vi "CSM - Remove Module in Boradcast Registry.vi"(0 "CSM Name":string, 11 "Error in":errorcluster caption="Error in (no error)") -> (4 "CSM Name(dup)":string, 15 "Error out":errorcluster)   [LabVIEW 2017, in "Communicable State Machine.lvlib"]
doc: "-- <b>输入控件</b> --\n- <b>CSM Name</b>:\n\n- <B>error in</B> can accept error information wired from VIs previously called. Use this information to decide if any functionality should be bypassed in the event of errors from other VIs.\n\nRight-click the <B>error in</B> control on the front panel and select <B>Explain Error</B> or <B>Explain Warning</B> from the shortcut menu for more information about the error.\n\n-- <b>输出控件</b> --\n- <b>CSM Name(dup)</b>:\n\n- <b>Error out</b>:\n- <B>error out</B> passes error or warning information out of a VI to be used by other VIs.\n\nRight-click the <B>error out</B> indicator on the front panel and select <B>Explain Error</B> or <B>Explain Warning</B> from the shortcut menu for more information about the error."
uses:
  Communicable State Machine.lvlib
  _Support/FGV-BroadcastRegistry/Operation-BroadcastRegistry.ctl
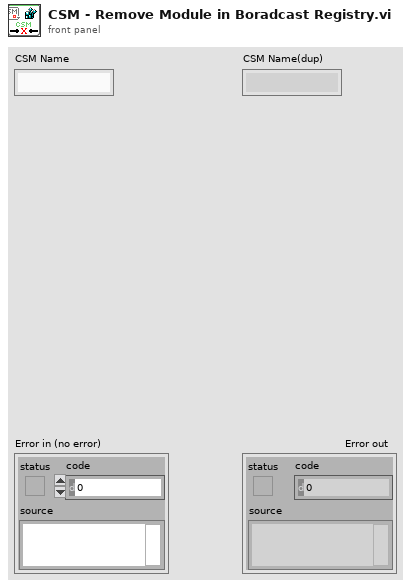
[diagram p1: front panel]
types:
  T1 = typedef "Communicable State Machine.lvlib/Operation-BroadcastRegistry.ctl" = enum16{"Delete Source Module", "Delete Target Module", "Remove Module", "Register", "Unregister", "Check", "List Status", "List Entries"}
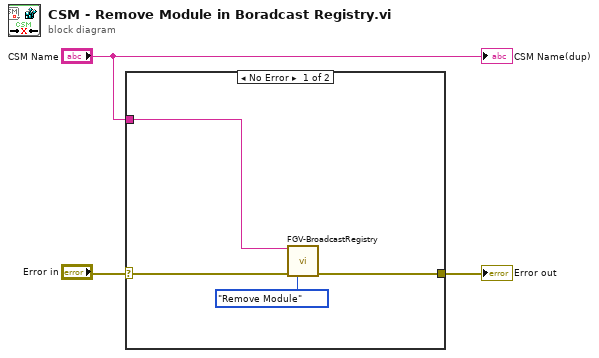
[diagram p0: block diagram]
diagram:
  n1 = case shown="No Error" "Error in" {
    selector: "Error in" -> [w6 w8]
    tunnel: [w5 w8] -> w2
    tunnel: "CSM Name" -> [w4 _]
    frame No Error {
      n2 = call "FGV-BroadcastRegistry.vi"("Source"=w4, "Error in"=w6, "Operation"=Operation-BroadcastRegistry."Remove Module") -> ("Error out"=w5:errorcluster)  [unwired: 11 in, 1 out]
    }
    frame Error {
    }
  }
  "Error out" <- w2
  "CSM Name(dup)" <- "CSM Name"
